vi "Filename increment.vi"(1 "TDMS filepath in":path, 3 "Added filename":string="COPY", 5 "error in (no error)":errorcluster) -> (15 "DUP TDMS filepath out":path, 16 "TDMS filepath increment":path, 18 "file or folder exists?":bool, 19 "error out":errorcluster)   [LabVIEW 2019, in "TDMS_DataHandler.lvclass"]
doc: "Creates a new filepath and name based on the number of files already present with the same name"
uses:
  TDMS_DataHandler.lvclass
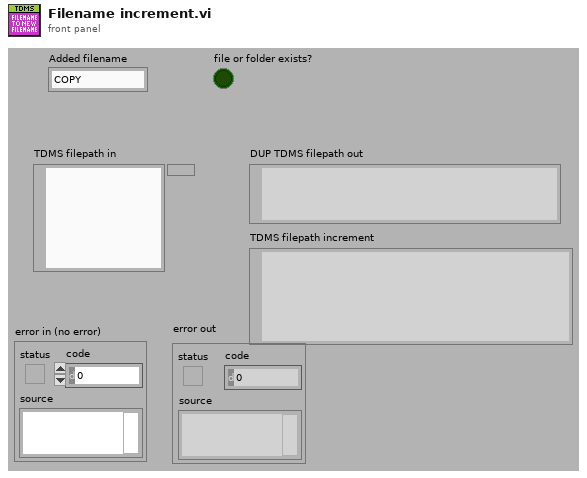
[diagram p1: front panel]
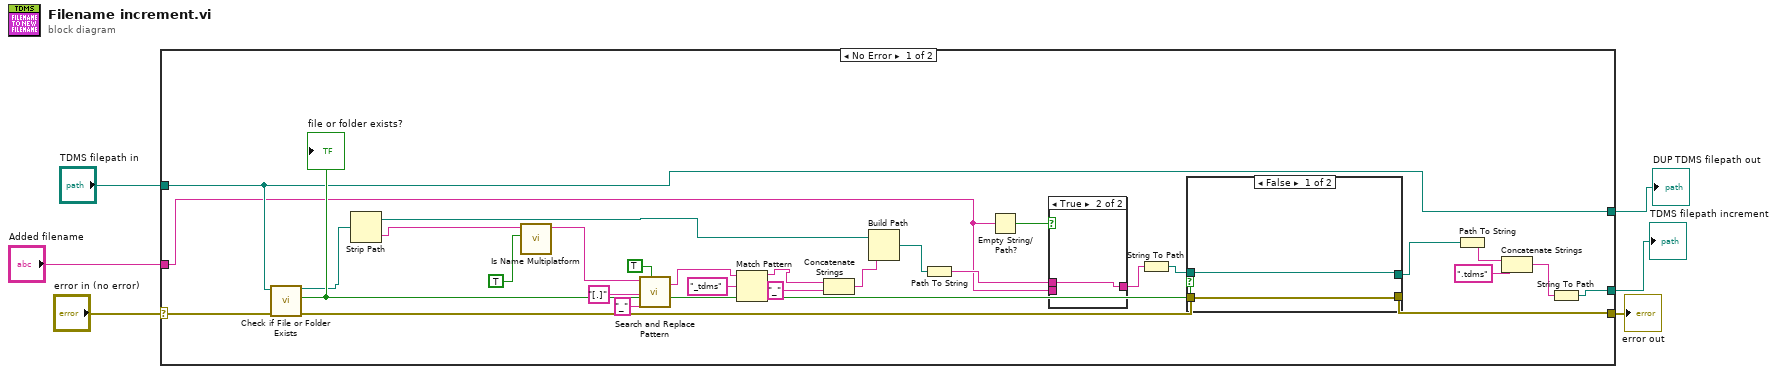
[diagram p0: block diagram]
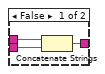
[diagram p2: hidden frame]
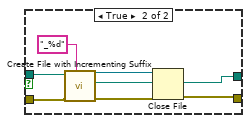
[diagram p3: hidden frame]
diagram:
  n1 = case shown="No Error" "error in (no error)" {
    selector: "error in (no error)" -> [w35 w49]
    tunnel: [w33 w49] -> w5
    tunnel: "TDMS filepath in" -> [w24 _]
    tunnel: [w24 _] -> w3
    tunnel: [w14 _] -> w2
    tunnel: "Added filename" -> [w8 _]
    frame No Error {
      n2 = call <vilib>:"Check if File or Folder Exists.vi"("error in (no error)"=w35, "path"=w24) -> ("error out"=w34:errorcluster, "file or folder exists?"=w32:bool, "dup path"=w31:path)  [unwired: 7 in]
      "file or folder exists?" <- w32
      n3 = Strip Path(path=w31) -> (stripped path=w29:path, name=w13:string)
      n4 = call <vilib>:"Is Name Multiplatform.vi"("filename must be valid on all platforms (F)"=TRUE, "filename"=w13) -> ("suggested filename"=w26:string)  [unwired: 5 in, 4 out]
      n5 = call <vilib>:"Search and Replace Pattern.vi"("string"=w26, "regular expression (\"\")"="[.]" ("regular expression (\"\")"), "replace string (\"\")"="_" ("replace string (\"\")"), "replace all? (F)"=TRUE) -> ("result string"=w23:string)  [unwired: 1 in, 1 out]
      n6 = Match Pattern(string=w23, regular expression="_tdms") -> (before substring=w21:string)  [unwired: 1 in, 3 out]
      n7 = Concatenate Strings(w21, "_" ("string")) -> (w19:string)
      n8 = Build Path(base path=w29, name or relative path=w19) -> (appended path=w12:path)
      n9 = Path To String(path=w12) -> (string=w11:string)
      n10 = Empty String/Path?(string/path=w8) -> (empty?=w7:bool)
      n11 = case shown="True" w7 {
        tunnel: w11 -> [w38 w39]
        tunnel: [w37 w39] -> w10
        tunnel: w8 -> [w36 _]
        frame False {
          n12 = Concatenate Strings(w38, w36) -> (w37:string)
        }
        frame True {
        }
      }
      n13 = String To Path(string=w10) -> (path=w9:path)
      n14 = case shown="False" w32 {
        tunnel: w34 -> [w41 w48]
        tunnel: [w41 w42] -> w33
        tunnel: w9 -> [w40 w46]
        tunnel: [w40 w45] -> w18
        frame False {
        }
        frame True {
          n15 = call <vilib>:"Create File with Incrementing Suffix.vi"("format string (\" (%d)\")"="_%d" ("format string (\" (%d)\")"), "error in (no error)"=w48, "file path"=w46) -> ("error out"=w43:errorcluster, "actual path"=w45:path, "refnum out"=w44:refnum<file>)  [unwired: 6 in]
          n16 = Close File(refnum=w44, error in=w43) -> (error out=w42:errorcluster)  [unwired: 1 out]
        }
      }
      n17 = Path To String(path=w18) -> (string=w17:string)
      n18 = Concatenate Strings(w17, ".tdms" ("string")) -> (w15:string)
      n19 = String To Path(string=w15) -> (path=w14:path)
    }
    frame Error {
    }
  }
  "error out" <- w5
  "DUP TDMS filepath out" <- w3
  "TDMS filepath increment" <- w2
